vi "Egi2_Pitch_Roll_Yaw_Rate_Set_Get.vi"(0 "Egi2 Yaw Rate Valid":u16, 1 "Egi2 Roll Rate Valid":u16, 2 "message handle in 2":u64, 3 "Egi2 Roll Rate":dbl, 4 "Egi2 Pitch Rate Valid":u16, 5 "error in (no error)":errorcluster, 6 "message handle in 3":u64, 7 "message handle in1":u64, 8 "Egi2 Yaw Rate":dbl, 9 "Egi2 Pitch Rate":dbl) -> (10 "Egi2 Pitch Rate Value OLD":u32 format="%.0b", 11 "Egi2 Pitch Rate Range Message":string, 12 "Egi2 Pitch Rate Value NEW":u32 format="%08b", 13 "Egi2 Roll Rate Range Message":string, 14 "Egi2 Roll Rate Value OLD":u32 format="%.0b", 15 "Egi2 Roll Rate Value NEW":u32 format="%08b", 16 "Egi2 Yaw Rate Value OLD":u32 format="%08b", 17 "Egi2 Yaw Rate Value NEW":u32 format="%08b", 18 "Egi2 Yaw Rate Range Message":string, 19 "error out":errorcluster)   [LabVIEW 2023]
uses:
  <instrlib>/BTI429Lib/Private/Utility/Get BNR Data.vi
  <instrlib>/BTI429Lib/Private/Utility/Set BNR Data.vi
  <instrlib>/BTI429Lib/Private/Utility/Set BNR SSM.vi
  <instrlib>/BTI429Lib/BTI429LV.lvlib
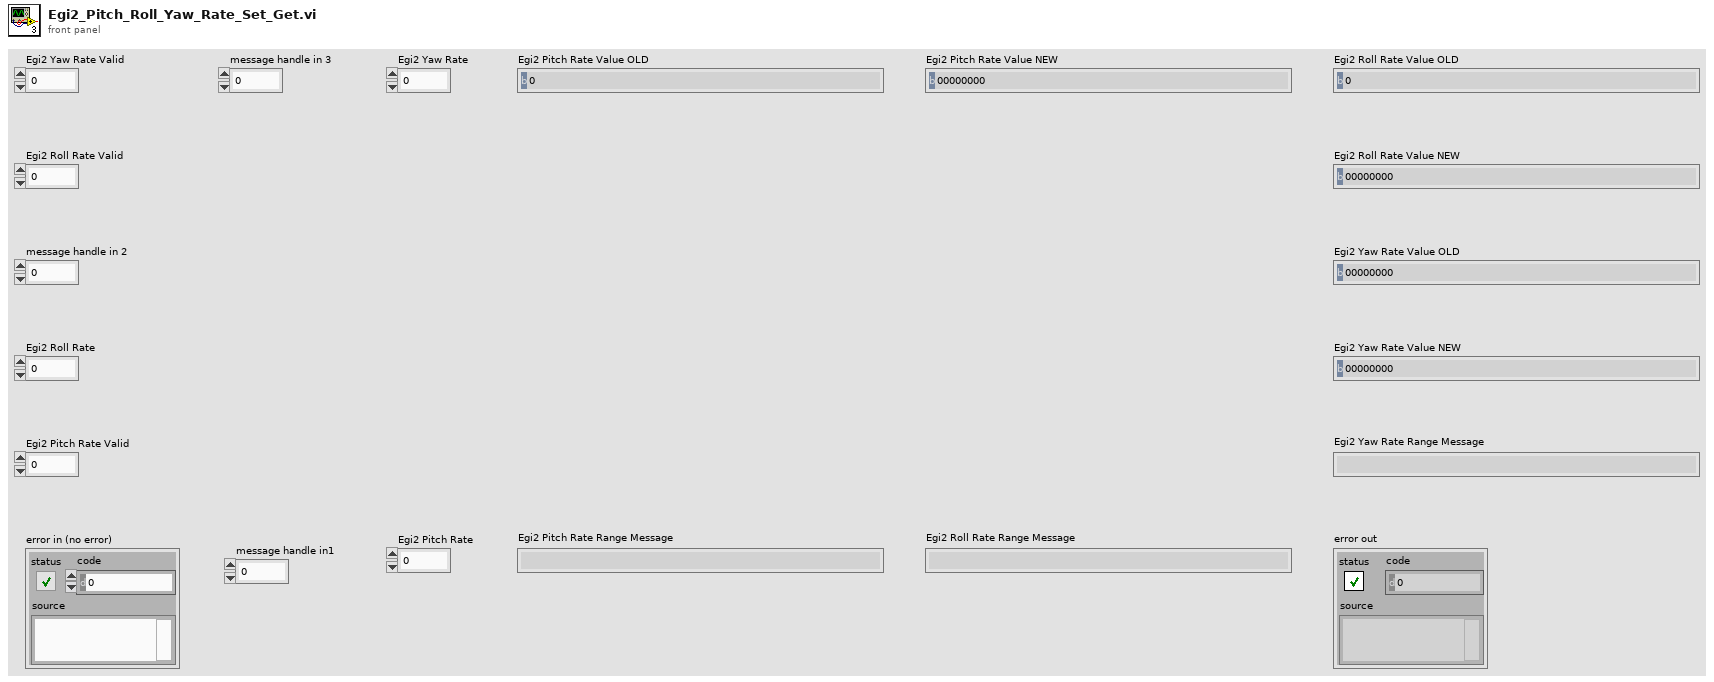
[diagram p1: front panel]
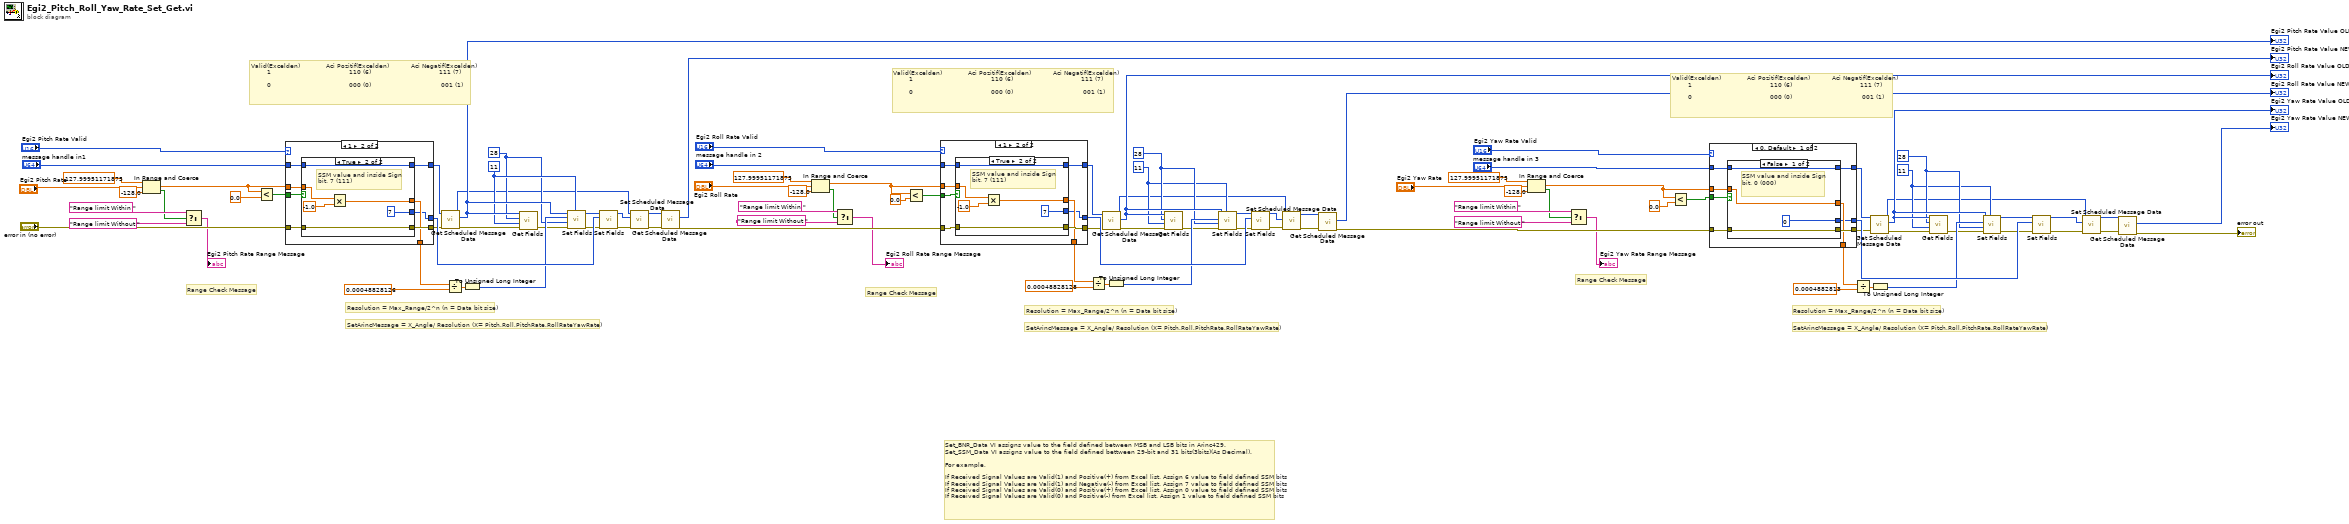
[diagram p0: block diagram]
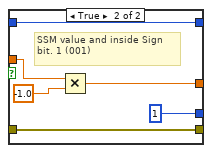
[diagram p2: hidden frame]
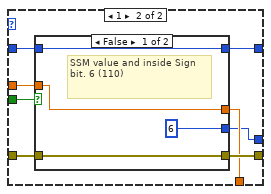
[diagram p3: hidden frame]
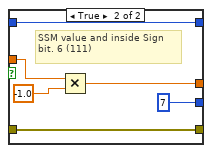
[diagram p4: hidden frame]
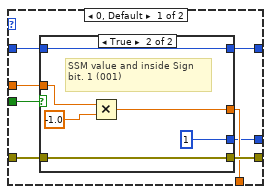
[diagram p5: hidden frame]
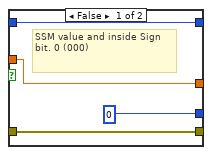
[diagram p6: hidden frame]
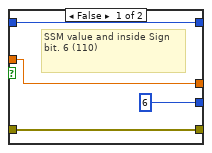
[diagram p7: hidden frame]
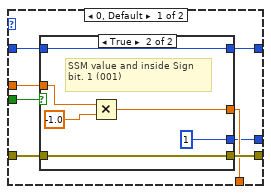
[diagram p8: hidden frame]
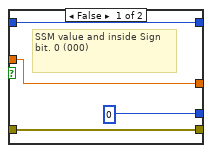
[diagram p9: hidden frame]
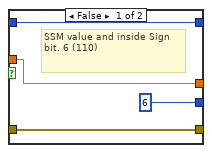
[diagram p10: hidden frame]
diagram:
  w6 = u16 28 ("most significant bit")
  w5 = u16 11 ("least significant bit")
  w27 = u16 28 ("most significant bit")
  w26 = u16 11 ("least significant bit")
  w18 = u16 28 ("most significant bit")
  w19 = u16 11 ("least significant bit")
  # "Range Check Message"
  # "SetArincMessage = X_Angle/ Resolution (X= Pitch,Roll,PitchRate,RollRateYawRate)"
  # "Resolution = Max_Range/2^n (n = Data bit size)"
  # "Range Check Message"
  # "Range Check Message"
  # "SetArincMessage = X_Angle/ Resolution (X= Pitch,Roll,PitchRate,RollRateYawRate)"
  # "Resolution = Max_Range/2^n (n = Data bit size)"
  # "SetArincMessage = X_Angle/ Resolution (X= Pitch,Roll,PitchRate,RollRateYawRate)"
  # "Resolution = Max_Range/2^n (n = Data bit size)"
  # "Set_BNR_Data VI assigns value to the field defined between MSB and LSB bits in Arinc429.\nSet_SSM_Data VI assigns value to the field defined bettween 29-bit and 31 bits(3bits)(As Decimal).\n\nFor example,\n\nIf Received Signal Values are Valid(1) and Positive(+) from Excel list. Assign 6 value to field defined SSM bits\nIf Received Signal Values are Valid(1) and Negative(-) from Excel list. Assign 7 value to field defined SSM bits\nIf Received Signal Values are Valid(0) and Positive(+) from Excel list. Assign 0 value to field defined SSM bits\nIf Received Signal Values are Valid(0) and Positive(-) from Excel list. Assign 1 value to field defined SSM bits"
  # "Valid(Excelden)             Aci Pozitif(Excelden)           Aci Negatif(Excelden) \n        1                                       110 (6)                                  111 (7)\n\n        0                                       000 (0)                                   001 (1)"
  # "Valid(Excelden)             Aci Pozitif(Excelden)           Aci Negatif(Excelden) \n        1                                       110 (6)                                  111 (7)\n\n        0                                       000 (0)                                   001 (1)"
  # "Valid(Excelden)             Aci Pozitif(Excelden)           Aci Negatif(Excelden) \n        1                                       110 (6)                                  111 (7)\n\n        0                                       000 (0)                                   001 (1)"
  n1 = In Range and Coerce(upper limit=127.99951171875, x="Egi2 Pitch Rate", lower limit=-128.0) -> (coerced(x)=w66:dbl, In Range?=w42:bool)
  n2 = Select(t="Range limit Within ", s=w42, f="Range limit Without ") -> (s? t:f=→"Egi2 Pitch Rate Range Message":string)
  n3 = Less?(x=w66, y=0.0) -> (x < y?=w67:bool)
  n4 = case shown="1" "Egi2 Pitch Rate Valid" {
    tunnel: [w107 w126] -> w68
    tunnel: [w105 w125] -> w63
    tunnel: "error in (no error)" -> [w108 w124]
    tunnel: "message handle in1" -> [w106 w123]
    tunnel: w67 -> [w101 w122]
    tunnel: [w103 w121] -> w65
    tunnel: w66 -> [w104 w120]
    tunnel: [w102 w119] -> w73
    frame 0, Default {
      n5 = case shown="True" w101 {
        tunnel: w104 -> [w112 w114]
        tunnel: [w112 w117] -> w103
        tunnel: w106 -> [w111 w116]
        tunnel: w108 -> [w110 w115]
        tunnel: [w111 w116] -> w105
        tunnel: [w110 w115] -> w107
        tunnel: [u16 0 ("value") u16 1 ("value")] -> w102
        frame False {
          # "SSM value and inside Sign bit. 0 (000)"
        }
        frame True {
          # "SSM value and inside Sign bit. 1 (001)"
          n6 = Multiply(x=w114, y=-1.0) -> (x*y=w117:dbl)
        }
      }
    }
    frame 1 {
      n7 = case shown="True" w122 {
        tunnel: w120 -> [w130 w135]
        tunnel: [w130 w134] -> w121
        tunnel: w123 -> [w129 w133]
        tunnel: w124 -> [w128 w132]
        tunnel: [w129 w133] -> w125
        tunnel: [w128 w132] -> w126
        tunnel: [u16 6 ("value") u16 7 ("value")] -> w119
        frame False {
          # "SSM value and inside Sign bit. 6 (110)"
        }
        frame True {
          # "SSM value and inside Sign bit. 7 (111)"
          n8 = Multiply(x=w135, y=-1.0) -> (x*y=w134:dbl)
        }
      }
    }
  }
  n9 = call <instrlib>:"Get Scheduled Message Data.vi"("error in (no error)"=w68, "message handle in"=w63) -> ("error out"=w15:errorcluster, "value"=w33:u32, "message handle out"=w17:u64)  [unwired: 7 in]
  "Egi2 Pitch Rate Value OLD" <- w33
  n10 = Divide(x=w65, y=0.00048828126) -> (x/y=w22:dbl)
  n11 = To Unsigned Long Integer(number=w22) -> (unsigned 32bit integer=w28:u32)
  n12 = call-poly <instrlib>:"Get Fields.vi"("error in (no error)"=w15, "least significant bit"=w19, "most significant bit"=w18, "message"=w33) -> ("error out"=w16:errorcluster)  [unwired: 6 in, 1 out]
  n13 = call-poly <instrlib>:"Set Fields.vi"("least significant bit"=w19, "error in (no error)"=w16, "most significant bit"=w18, "value"=w28, "message"=w33) -> ("error out"=w69:errorcluster, "message out"=w72:u32)  [unwired: 5 in]
  n14 = call-poly <instrlib>:"Set Fields.vi"("error in (no error)"=w69, "value"=w73, "message"=w72) -> ("error out"=w70:errorcluster, "message out"=w71:u32)  [unwired: 7 in]
  n15 = call <instrlib>:"Set Scheduled Message Data.vi"("error in (no error)"=w70, "value"=w71, "message handle in"=w17) -> ("error out"=w38:errorcluster, "message handle out"=w39:u64)  [unwired: 7 in]
  n16 = call <instrlib>:"Get Scheduled Message Data.vi"("error in (no error)"=w38, "message handle in"=w39) -> ("error out"=w77:errorcluster, "value"=→"Egi2 Pitch Rate Value NEW":u32)  [unwired: 7 in, 1 out]
  n17 = In Range and Coerce(upper limit=127.99951171875, x="Egi2 Roll Rate", lower limit=-128.0) -> (coerced(x)=w75:dbl, In Range?=w49:bool)
  n18 = Select(t="Range limit Within ", s=w49, f="Range limit Without ") -> (s? t:f=→"Egi2 Roll Rate Range Message":string)
  n19 = Less?(x=w75, y=0.0) -> (x < y?=w76:bool)
  n20 = case shown="1" "Egi2 Roll Rate Valid" {
    tunnel: [w143 w162] -> w79
    tunnel: [w139 w161] -> w80
    tunnel: w77 -> [w144 w160]
    tunnel: "message handle in 2" -> [w138 w159]
    tunnel: w76 -> [w137 w158]
    tunnel: [w141 w157] -> w78
    tunnel: w75 -> [w142 w156]
    tunnel: [w140 w155] -> w85
    frame 0, Default {
      n21 = case shown="True" w137 {
        tunnel: w142 -> [w148 w150]
        tunnel: [w148 w153] -> w141
        tunnel: w138 -> [w147 w152]
        tunnel: w144 -> [w146 w151]
        tunnel: [w147 w152] -> w139
        tunnel: [w146 w151] -> w143
        tunnel: [u16 0 ("value") u16 1 ("value")] -> w140
        frame False {
          # "SSM value and inside Sign bit. 0 (000)"
        }
        frame True {
          # "SSM value and inside Sign bit. 1 (001)"
          n22 = Multiply(x=w150, y=-1.0) -> (x*y=w153:dbl)
        }
      }
    }
    frame 1 {
      n23 = case shown="True" w158 {
        tunnel: w156 -> [w166 w171]
        tunnel: [w166 w170] -> w157
        tunnel: w159 -> [w165 w169]
        tunnel: w160 -> [w164 w168]
        tunnel: [w165 w169] -> w161
        tunnel: [w164 w168] -> w162
        tunnel: [u16 6 ("value") u16 7 ("value")] -> w155
        frame False {
          # "SSM value and inside Sign bit. 6 (110)"
        }
        frame True {
          # "SSM value and inside Sign bit. 7 (111)"
          n24 = Multiply(x=w171, y=-1.0) -> (x*y=w170:dbl)
        }
      }
    }
  }
  n25 = Divide(x=w78, y=0.00048828128) -> (x/y=w31:dbl)
  n26 = call <instrlib>:"Get Scheduled Message Data.vi"("error in (no error)"=w79, "message handle in"=w80) -> ("error out"=w24:errorcluster, "value"=w34:u32, "message handle out"=w23:u64)  [unwired: 7 in]
  "Egi2 Roll Rate Value OLD" <- w34
  n27 = To Unsigned Long Integer(number=w31) -> (unsigned 32bit integer=w32:u32)
  n28 = call-poly <instrlib>:"Get Fields.vi"("error in (no error)"=w24, "least significant bit"=w26, "most significant bit"=w27, "message"=w34) -> ("error out"=w25:errorcluster)  [unwired: 6 in, 1 out]
  n29 = call-poly <instrlib>:"Set Fields.vi"("least significant bit"=w26, "error in (no error)"=w25, "most significant bit"=w27, "value"=w32, "message"=w34) -> ("error out"=w81:errorcluster, "message out"=w84:u32)  [unwired: 5 in]
  n30 = call-poly <instrlib>:"Set Fields.vi"("error in (no error)"=w81, "value"=w85, "message"=w84) -> ("error out"=w82:errorcluster, "message out"=w83:u32)  [unwired: 7 in]
  n31 = call <instrlib>:"Set Scheduled Message Data.vi"("error in (no error)"=w82, "value"=w83, "message handle in"=w23) -> ("error out"=w35:errorcluster, "message handle out"=w36:u64)  [unwired: 7 in]
  n32 = call <instrlib>:"Get Scheduled Message Data.vi"("error in (no error)"=w35, "message handle in"=w36) -> ("error out"=w86:errorcluster, "value"=→"Egi2 Roll Rate Value NEW":u32)  [unwired: 7 in, 1 out]
  n33 = In Range and Coerce(upper limit=127.99951171875, x="Egi2 Yaw Rate", lower limit=-128.0) -> (coerced(x)=w88:dbl, In Range?=w56:bool)
  n34 = Select(t="Range limit Within ", s=w56, f="Range limit Without ") -> (s? t:f=→"Egi2 Yaw Rate Range Message":string)
  n35 = Less?(x=w88, y=0.0) -> (x < y?=w87:bool)
  n36 = case shown="0, Default" "Egi2 Yaw Rate Valid" {
    tunnel: [w179 w198] -> w91
    tunnel: [w175 w197] -> w90
    tunnel: w86 -> [w180 w196]
    tunnel: "message handle in 3" -> [w174 w195]
    tunnel: w87 -> [w173 w194]
    tunnel: [w177 w193] -> w92
    tunnel: w88 -> [w178 w192]
    tunnel: [w176 w191] -> w97
    frame 0, Default {
      n37 = case shown="False" w173 {
        tunnel: w178 -> [w184 w186]
        tunnel: [w184 w189] -> w177
        tunnel: w174 -> [w183 w188]
        tunnel: w180 -> [w182 w187]
        tunnel: [w183 w188] -> w175
        tunnel: [w182 w187] -> w179
        tunnel: [u16 0 ("value") u16 1 ("value")] -> w176
        frame False {
          # "SSM value and inside Sign bit. 0 (000)"
        }
        frame True {
          # "SSM value and inside Sign bit. 1 (001)"
          n38 = Multiply(x=w186, y=-1.0) -> (x*y=w189:dbl)
        }
      }
    }
    frame 1 {
      n39 = case shown="False" w194 {
        tunnel: w192 -> [w202 w207]
        tunnel: [w202 w206] -> w193
        tunnel: w195 -> [w201 w205]
        tunnel: w196 -> [w200 w204]
        tunnel: [w201 w205] -> w197
        tunnel: [w200 w204] -> w198
        tunnel: [u16 6 ("value") u16 7 ("value")] -> w191
        frame False {
          # "SSM value and inside Sign bit. 6 (110)"
        }
        frame True {
          # "SSM value and inside Sign bit. 6 (111)"
          n40 = Multiply(x=w207, y=-1.0) -> (x*y=w206:dbl)
        }
      }
    }
  }
  n41 = Divide(x=w92, y=0.0004882813) -> (x/y=w9:dbl)
  n42 = call <instrlib>:"Get Scheduled Message Data.vi"("error in (no error)"=w91, "message handle in"=w90) -> ("error out"=w3:errorcluster, "value"=w11:u32, "message handle out"=w2:u64)  [unwired: 7 in]
  "Egi2 Yaw Rate Value OLD" <- w11
  n43 = To Unsigned Long Integer(number=w9) -> (unsigned 32bit integer=w10:u32)
  n44 = call-poly <instrlib>:"Get Fields.vi"("error in (no error)"=w3, "least significant bit"=w5, "most significant bit"=w6, "message"=w11) -> ("error out"=w4:errorcluster)  [unwired: 6 in, 1 out]
  n45 = call-poly <instrlib>:"Set Fields.vi"("least significant bit"=w5, "error in (no error)"=w4, "most significant bit"=w6, "value"=w10, "message"=w11) -> ("error out"=w93:errorcluster, "message out"=w96:u32)  [unwired: 5 in]
  n46 = call-poly <instrlib>:"Set Fields.vi"("error in (no error)"=w93, "value"=w97, "message"=w96) -> ("error out"=w94:errorcluster, "message out"=w95:u32)  [unwired: 7 in]
  n47 = call <instrlib>:"Set Scheduled Message Data.vi"("error in (no error)"=w94, "value"=w95, "message handle in"=w2) -> ("error out"=w12:errorcluster, "message handle out"=w13:u64)  [unwired: 7 in]
  n48 = call <instrlib>:"Get Scheduled Message Data.vi"("error in (no error)"=w12, "message handle in"=w13) -> ("error out"=→"error out":errorcluster, "value"=→"Egi2 Yaw Rate Value NEW":u32)  [unwired: 7 in, 1 out]
